vi "Meas_global.vi"() -> ()   [LabVIEW 2015]
uses:
  Controls/Ch_and_Spans.ctl
  Controls/Graph_Type.ctl
  Controls/Post_Process.ctl
  Controls/Trigger_Mode.ctl
  Controls/PWA_Data.ctl
  Controls/Correlation_cluster1.ctl
  Controls/XY_Plot_Cluster.ctl
  Controls/Time_Trace_Cluster.ctl
  Controls/Analysis_info_cluster.ctl
  Controls/Inst_type.ctl
  Controls/Instrument_Array.ctl
  Controls/LDA_Setup.ctl
  Controls/Setup.ctl
panel:
  in  "Tab Control":T1(tab)
  out "Acq ready":bool
  out "Abs Press (mbar)":dbl=1005.0 format="%.2f"
  in  "Start Time of experiment":dbl format="%.2f"
  in  "Requested No of samples":i32=128 min=0 step=1
  out "Temp":dbl=20.0 format="%.1f"
  in  "Requested No of blocks":i32
  out "Actual Sampling rate (Hz)":dbl=1000.0 format="%.2f"
  in  "Post Process":T2
  out "Current Block No":i32
  in  "Remote control":bool
  in  "ADAM Ch Names":string[](array[string])
  in  "Processing last block?":bool
  in  "Averaging time (min)":dbl=6.0 format="%.2f"
  out "Actual Measurement time (min)":dbl=6.0 format="%.2f"
  in  "People to Email":string[](array[string])
  in  "Requested Sampling rate":dbl=100.0 format="%.2f"
  in  "Repeat Measurement?":bool
  in  "Blocks to Skip":i32[](array[numeric])
  out "No of Analogue Samples":i32=128 min=0 step=1
  in  "Iteration Number":i32
  out "OverrideWait":bool
  in  "setup":T3=enum."Show Setup"
  out "Flattened data type":enum16{"4.x", "Standard"}(ring)
  out "Time Data was Aquired":dbl format="%.2f"
  in  "Meas Setup filename":string
  in  "Extra Comments":string
  out "ProgRevisionInfo":string
  in  "New Setup String":string
  in  "Pre Setup String":string
  in  "Comments":string
  in  "Raw data file":path
  in  "File":T4(ring)
  in  "Results file":path
  out "Raw data option":enum16{"Save raw data", "Raw data not saved"}(ring)
  out "Start of I16 data (bytes)":i32
  out "Calib file strings":string[](array[string])
  out "Calib type name":string[](array[string])
  out "DAQ Error":errorcluster
  in  "Acquisition vi to Run":string
  in  "Analogue volts":dbl[][](array[numeric]) format="%.2f"
  in  "input terminal configuration":i32(ring)=10106 items=["default"=-1, "RSE"=10083, "NRSE"=10078, "Differential"=10106, "Pseudodifferential"=12529]
  in  "Trigger mode":T5
  in  "Continuous time trace?":bool
  in  "Analogue data":enum16{"No Analogue data", "Take Analogue data"}(ring)
  in  "Time Continuous Across Blocks":bool
  in  "output polarity":u16(ring)=1 items=["do not change", "positive", "negative"]
  in  "Over/Under string":string
  out "Ch & spans + mod limits":T6[](array[typedef]) {"low limit (-10V)" format="%.3f"; "high limit (10V)" format="%.3f"}
  out "Ch & spans":T6[](array[typedef]) {"low limit (-10V)" format="%.3f"; "high limit (10V)" format="%.3f"}
  in  "LDA set up":T7={"dimensions"=enum."2D", "Analogue Freq Multiplier"=0.1} {"Analogue Freq Multiplier" min=0.1 max=100.0 format="%_5g"}
  in  "Analogue Sampling Rate":dbl
  in  "No of Non Analogue Chs":i32
  in  "PWA Data":T8
  in  "stop":bool
  in  "No of Vari Spaced Chs":i32
  in  "LDA frequency":dbl
  in  "BSA data rate string":string
  in  "LDA data":enum16{"No LDA data", "Take LDA data"}(ring)
  in  "Synchronise with LDA":bool
  in  "No of LDA data channels":i32
  in  "Data Validity":dbl=3.0 min=1.0 max=10.0 format="%.2f"
  in  "Duplicate channels":i32[](array[numeric])
  in  "Smoothing setups":T9(array[cluster]) {"Y axis"."Format" items=["Decimal", "Scientific", "Engineering"]; "Y axis"."Mapping" items=["Linear", "Logarithmic"]; "X axis"."Format" items=["Decimal", "Scientific", "Engineering"]; "X axis"."Mapping" items=["Linear", "Logarithmic"]}
  in  "Cross wire + or -ve":T10(ring)
  in  "Second Graph":T12={"Plot 1"=1, "Plot 2"=3, "Save graph"=0, "Plot Type"=enum."Voltage trace"} {"Save graph" items=["Do not save plot", "Save plot"]; "Plot 2" items=["Nothing", "Velocity1", "Arr time1", "Velocity2", "Arr time2"]; "Plot 1" items=["Nothing", "Velocity1", "Arr time1", "Velocity2", "Arr time2"]}
  in  "First Graph":T12={"Plot 1"=1, "Plot 2"=3, "Save graph"=0, "Plot Type"=enum."Voltage trace"} {"Save graph" items=["Do not save plot", "Save plot"]; "Plot 2" items=["Nothing", "Velocity1", "Arr time1", "Velocity2", "Arr time2"]; "Plot 1" items=["Nothing", "Velocity1", "Arr time1", "Velocity2", "Arr time2"]}
  in  "No of bins in histogram":i32
  in  "correlate":i32[][](array[numeric]) min=0 max=8
  in  "Insts for plotting":u16[][](array[ring]) items=["Nothing", "Ref Prop 1", "XW1 1", "XW2 1"]
  in  "Analysis Info cluster":T13[](array[typedef]) {"Sd Error in Variance" format="%.2f"; "Skew_u" format="%.2f"; "% u'/U" format="%.2f"; "Sd Error in Mean" format="%.2f"; "Kurt_u" format="%.2f"; "u^4" format="%.2f"; "u^3" format="%.2f"; "U" format="%.2f"; "u^2" format="%.2f"}
  in  "Time Trace":T16[](array[typedef])
  in  "Autocorrelation":T17[](array[typedef])
  in  "Histogram":T17[](array[typedef])
  in  "Spectra":T17[](array[typedef])
  in  "Correlation Results":T18[](array[typedef]) {"u^2w^2" format="%.2f"; "u^3w" format="%.2f"; "uw^3" format="%.2f"; "uw/u'w'" format="%.2f"; "uw^2" format="%.2f"; "u^2w" format="%.2f"; "uw" format="%.2f"}
  in  "Error Messages":string
  out "Diagnostic info":string[][](table)
  out "Vel stat display":string[][](table)
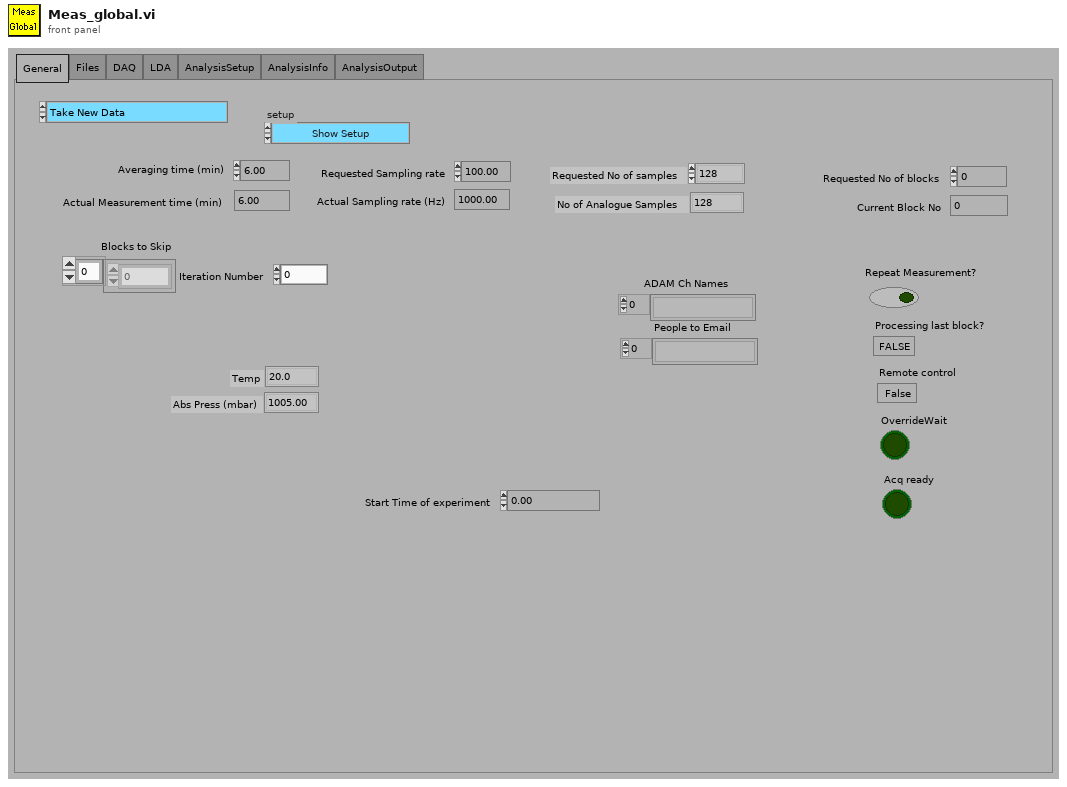
[diagram p1: front panel]
types:
  T1 = enum32{"General", "Files", "DAQ", "LDA", "AnalysisSetup", "AnalysisInfo", "AnalysisOutput"}
  T2 = typedef "Post_Process.ctl" = enum16{"Take New Data", "Post Process Raw Data File"}
  T3 = typedef "Setup.ctl" = enum16{"Run Program", "Show Setup", "Save Current Setup", "Setup Front Panel"}
  T4 = enum16{"Save no data", "Save data in new files", "Save data in existing files"}
  T5 = typedef "Trigger_Mode.ctl" = enum16{"Free Running", "Start on Trigger", "Trigger Every Block", "Trigger Every Sample"}
  T6 = typedef "Ch_and_Spans.ctl" = cluster{"high limit (10V)":sgl, "low limit (-10V)":sgl, "Ch No":i16, "Var name":string, "Use Latest Calib":bool}
  T7 = typedef "LDA_Setup.ctl" = cluster{"dimensions":enum16{"1D", "2D"}, "Analogue Freq Multiplier":dbl}
  T8 = typedef "PWA_Data.ctl" = enum16{"No PWA Data", "One Ch PWA"}
  T9 = cluster{"Start Index":i32, "End Index":i32, "Smoothing":enum16{"Linear", "Logarithmic"}, "Number of smoothed estimates":i32, "X axis":cluster{"Mapping":u16, "Format":u16}, "Y axis":cluster{"Mapping":u16, "Format":u16}, "Use Whole Input Array?":bool}[]
  T10 = enum16{"2nd component as calculated", "2nd component multipled by -1"}
  T11 = typedef "Graph_Type.ctl" = enum16{"Show no graph", "Voltage trace", "Velocity trace", "Vel histogram", "Spectrum", "f.E(f) v Log f", "Auto-Corr"}
  T12 = cluster{"Plot 1":u16, "Plot 2":u16, "Save graph":u16, "Plot Type":T11}
  T13 = typedef "Analysis_info_cluster.ctl" = cluster{"Colour":u32, "Inst type":T14, "Inst name":string, "Symbol":string, "Code name":string, "Extra Info":string, "Inst Array":T15, "Extra Titles":string[], "Extra Values":string[], "U":dbl, "u^2":dbl, "u^3":dbl, "u^4":dbl, "Skew_u":dbl, "Kurt_u":dbl, "Sd Error in Mean":dbl, "% u'/U":dbl, "X":dbl, "Y":dbl, "Z":dbl, "Timescale integral to 25%":dbl, "Sd Error in Variance":dbl, "Calib File":path, "Calib Constants":dbl[], "Output Position":bool, "Full Stats":bool, "Av Sampling Rate":dbl, "Av No of Samples":dbl, "Total Meas Time (s)":dbl, "ADAM Ch Name":string}
  T14 = typedef "Inst_type.ctl" = enum16{"Propeller anemometer", "Raw voltage", "Pressure Transducer", "Pitot-static tube", "Preston tube", "Hot wire", "Cross wire 1", "Cross wire 2", "Generic Linear", "Generic Polynomial", "Generic BackPoly", "Fast FID", "Thermocouple", "Cold wire", "Pulsed Wire", "LDA Vel", "LDA Tran time", "LDA Arr time", "Microphone"}
  T15 = typedef "Instrument_Array.ctl" = enum16{"PWA", "LDA", "Analogue"}
  T16 = typedef "Time_Trace_Cluster.ctl" = cluster{"Weighting":dbl[], "Time (s)":dbl[], "Voltage":dbl[], "Eng Values":dbl[]}
  T17 = typedef "XY_Plot_Cluster.ctl" = cluster{"First Name":string, "Second Name":string, "X axis name":string, "Y axis name":string, "X array":dbl[], "Y array":dbl[]}
  T18 = typedef "Correlation_cluster1.ctl" = cluster{"U inst":string, "uw":dbl, "u^2w":dbl, "uw^2":dbl, "uw/u'w'":dbl, "W inst":string, "uw^3":dbl, "u^3w":dbl, "u^2w^2":dbl, "Index U":i32, "Index W":i32}
diagram:
